vi "Stop Work.vi"(6 "Controller name":string, 8 "error in (no error)":errorcluster, 9 "Reply":bool=TRUE, 10 "Reply to":refnum<class "Stop Response Msg.lvclass">, 11 "Worker in":refnum<class "Worker Actor.lvclass">) -> (0 "error out":errorcluster, 3 "Worker out":refnum<class "Worker Actor.lvclass">)   [LabVIEW 2021, in "Worker Actor.lvclass"]
uses:
  Worker Actor.lvclass
  C:/GitHub/LabActor/Template Module/Template Module.lvclass
  Controllers/Process Controller Messages/Stop Response Msg/Stop Response Msg.lvclass
  NHMFL_Core/Libraries/Instruments/Instrument Driver/Worker State.ctl
  Worker Actor.lvclass/Worker Actor.ctl
  Template Module/Template Module.lvclass/Template Module.ctl
  Controllers/Process Controller Messages/Stop Response Msg/Stop Response Msg.lvclass/Stop Response Msg.ctl
  Controllers/Process Controller Messages/Stop Response Msg/Write Name.vi
  Template Module/Write State.vi
  Template Module/Read Name.vi
  Write Pause requested.vi
  Write Paused.vi
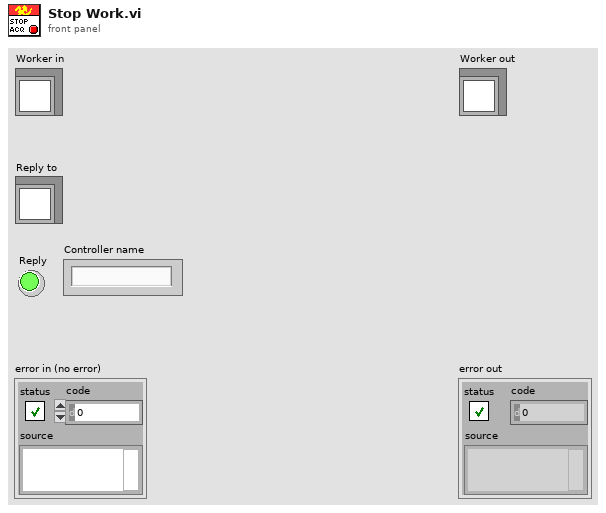
[diagram p1: front panel]
types:
  T1 = typedef "Worker State.ctl" = enum16{"Idle", "Starting", "Working", "Stopping"}
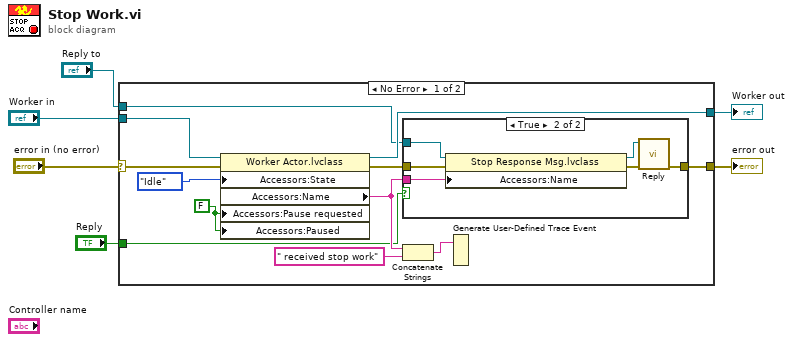
[diagram p0: block diagram]
diagram:
  n1 = case shown="No Error" "error in (no error)" {
    selector: "error in (no error)" -> [w16 w27]
    tunnel: [w9 w27] -> w5
    tunnel: [w17 w26] -> w3
    tunnel: "Worker in" -> [w18 w26]
    tunnel: "Reply to" -> [w12 _]
    tunnel: "Reply" -> [w8 _]
    frame No Error {
      w7 = FALSE ("Pause requested")
      n2 = property class="Worker Actor.lvclass"(reference=w18, error in=w16, "Accessors:State"=Worker_State."Idle" ("State"), "Accessors:Pause requested"=w7, "Accessors:Paused"=w7) -> (reference out=w17:refnum<class "Worker Actor.lvclass">, error out=w10:errorcluster, "Accessors:Name"=w11:string)
      n3 = case shown="True" w8 {
        tunnel: w12 -> [_ w25]
        tunnel: w11 -> [_ w24]
        tunnel: w10 -> [w19 w23]
        tunnel: [w19 w20] -> w9
        frame False {
        }
        frame True {
          n4 = property class="Stop Response Msg.lvclass"(reference=w25, error in=w23, "Accessors:Name"=w24) -> (reference out=w22:refnum<class "Stop Response Msg.lvclass">, error out=w21:errorcluster)
          n5 = call-dynamic "Reply.vi"("error in (no error)"=w21, "Self-addressed Msg in"=w22) -> ("error out"=w20:errorcluster)  [unwired: 8 in, 1 out]
        }
      }
      n6 = Concatenate Strings(w11, " received stop work" ("string")) -> (w14:string)
      n7 = Generate User-Defined Trace Event(2:w14) -> ()  [unwired: 1 in]
    }
    frame Error {
    }
  }
  "error out" <- w5
  "Worker out" <- w3
